vi "decode point message.vi"(11 "input stream":u8) -> (2 "new y":bool=TRUE, 3 "new x":bool=TRUE, 4 "waiting for new message":bool, 5 "decoder state":T1)   [LabVIEW 2010]
uses:
  vision decoder state typedef.ctl
  Deleteme/line driveable paths global.vi
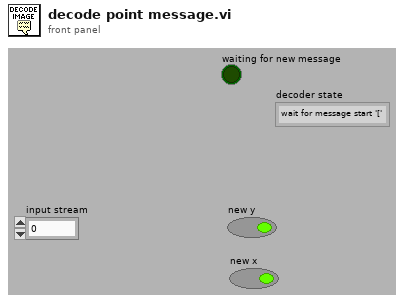
[diagram p1: front panel]
types:
  T1 = typedef "vision decoder state typedef.ctl" = enum16{"wait for message start '['", "wait for point start '(' ", "record x value", "record y value", "scan complete"}
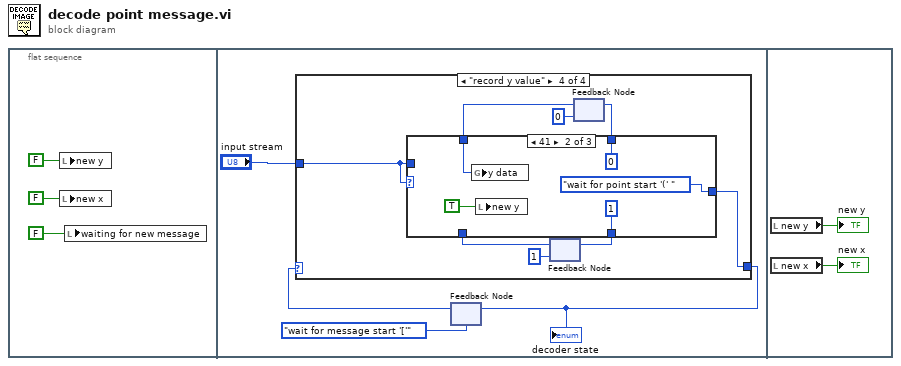
[diagram p0: block diagram]
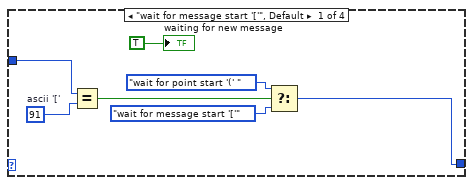
[diagram p2: hidden frame]
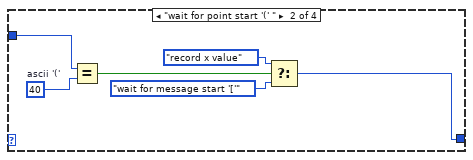
[diagram p3: hidden frame]
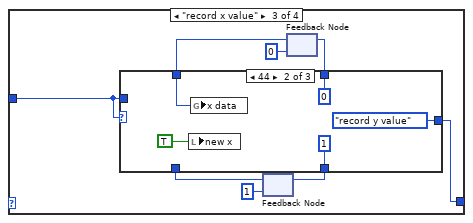
[diagram p4: hidden frame]
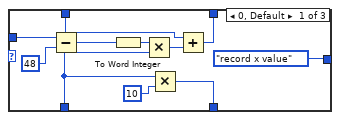
[diagram p5: hidden frame]
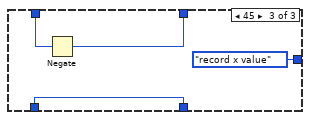
[diagram p6: hidden frame]
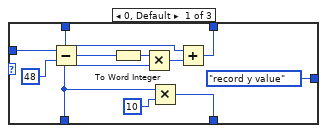
[diagram p7: hidden frame]
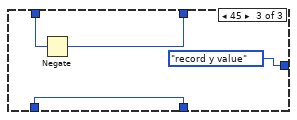
[diagram p8: hidden frame]
diagram:
  n1 = flat-sequence {
    frame #0 {
      n2 = local write "new y"(FALSE) -> ()
      n3 = local write "new x"(FALSE) -> ()
      n4 = local write "waiting for new message"(FALSE) -> ()
    }
    frame #1 {
      n5 = feedback #1(vision_decoder_state_typedef."wait for message start '['" ("Enum")) -> (w6:T1)
      n6 = case shown="\"record y value\"" w6 {
        tunnel: "input stream" -> [w13 w19 w22 w50]
        tunnel: [w9 w15 w21 w49] -> w4
        frame "wait for message start '['", Default {
          w14 = u8 91  # ascii '['
          n7 = Equal?(x=w13, y=w14) -> (x = y?=w12:bool)
          n8 = Select(t=vision_decoder_state_typedef."wait for point start '(' " ("Enum"), s=w12, f=vision_decoder_state_typedef."wait for message start '['" ("Enum")) -> (s? t:f=w9:T1)
          "waiting for new message" <- TRUE ("waiting for new message")
        }
        frame "wait for point start '(' " {
          w20 = u8 40  # ascii '('
          n9 = Equal?(x=w19, y=w20) -> (x = y?=w18:bool)
          n10 = Select(t=vision_decoder_state_typedef."record x value" ("Enum"), s=w18, f=vision_decoder_state_typedef."wait for message start '['" ("Enum")) -> (s? t:f=w15:T1)
        }
        frame "record x value" {
          n11 = feedback #2(i16 1) -> (w26:i16)
          n12 = feedback #3(i16 0) -> (w23:i16)
          n13 = case shown="44" w22 {
            tunnel: w22 -> [w39 _ _]
            tunnel: [w35 i16 1 w45] -> w28
            tunnel: w26 -> [w34 _ w45]
            tunnel: [w31 i16 0 w46] -> w25
            tunnel: w23 -> [w30 w40 w48]
            tunnel: [vision_decoder_state_typedef."record x value" ("Enum") vision_decoder_state_typedef."record y value" ("Enum") vision_decoder_state_typedef."record x value" ("Enum")] -> w21
            frame 0, Default {
              n14 = Subtract(x=w39, y=u8 48) -> (x-y=w37:u8)
              n15 = To Word Integer(number=w37) -> (16bit integer=w33:i16)
              n16 = Multiply(x=w33, y=w34) -> (x*y=w32:i16)
              n17 = Multiply(x=w34, y=i16 10) -> (x*y=w35:i16)
              n18 = Add(x=w30, y=w32) -> (x+y=w31:i16)
            }
            frame 44 {
              n19 = local write "new x"(TRUE) -> ()
              n20 = global write "line driveable paths global.vi" "x data"(w40) -> ()
            }
            frame 45 {
              n21 = Negate(x=w48) -> (-x=w46:i16)
            }
          }
          n22 = feedback-in #2(w28) -> ()
          n23 = feedback-in #3(w25) -> ()
        }
        frame "record y value" {
          n24 = feedback #4(i16 1) -> (w54:i16)
          n25 = feedback #5(i16 0) -> (w51:i16)
          n26 = case shown="41" w50 {
            tunnel: w50 -> [w67 _ _]
            tunnel: [w63 i16 1 w73] -> w56
            tunnel: w54 -> [w62 _ w73]
            tunnel: [w59 i16 0 w74] -> w53
            tunnel: w51 -> [w58 w68 w76]
            tunnel: [vision_decoder_state_typedef."record y value" ("Enum") vision_decoder_state_typedef."wait for point start '(' " ("Enum") vision_decoder_state_typedef."record y value" ("Enum")] -> w49
            frame 0, Default {
              n27 = Subtract(x=w67, y=u8 48) -> (x-y=w65:u8)
              n28 = To Word Integer(number=w65) -> (16bit integer=w61:i16)
              n29 = Multiply(x=w61, y=w62) -> (x*y=w60:i16)
              n30 = Multiply(x=w62, y=i16 10) -> (x*y=w63:i16)
              n31 = Add(x=w58, y=w60) -> (x+y=w59:i16)
            }
            frame 41 {
              n32 = global write "line driveable paths global.vi" "y data"(w68) -> ()
              n33 = local write "new y"(TRUE) -> ()
            }
            frame 45 {
              n34 = Negate(x=w76) -> (-x=w74:i16)
            }
          }
          n35 = feedback-in #4(w56) -> ()
          n36 = feedback-in #5(w53) -> ()
        }
      }
      "decoder state" <- w4
      n37 = feedback-in #1(w4) -> ()
    }
    frame #2 {
      n38 = local read "new y"() -> (→"new y":bool)
      n39 = local read "new x"() -> (→"new x":bool)
    }
  }
